vi "Init Events.vi"(8 "error in (no error)":errorcluster, 11 "DbgTimers in":refnum<class "DbgTimers.lvclass">) -> (0 "error out":errorcluster, 3 "DbgTimers out":refnum<class "DbgTimers.lvclass">)   [LabVIEW 2017, in "DbgTimers.lvclass"]
doc: "Developed by Kevin Thompson\nkevin@thompsonengineering.net\n\nCopyright 2018-2020\nThompson Engineering, LLC"
uses:
  DbgTimers.lvclass
  Ichor_Common/DataTypes/TD Async CmdMsg EventData--cluster.ctl
  DbgTimers.lvclass/DbgTimers.ctl
  Accessors/Get PublicEvents.vi
  Accessors/Set PublicEvents.vi
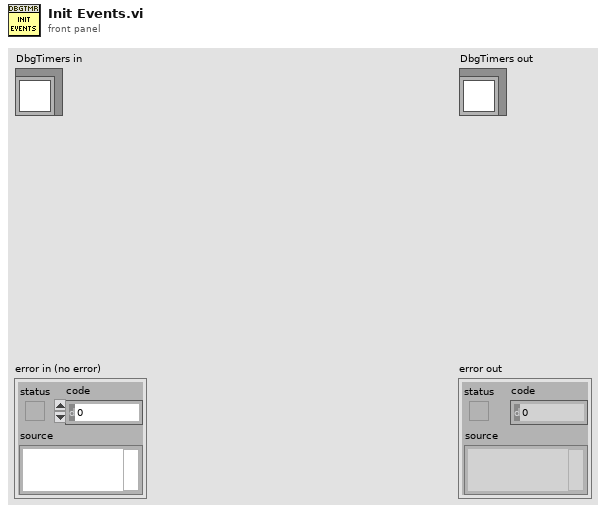
[diagram p1: front panel]
types:
  T1 = typedef "TD Async CmdMsg EventData--cluster.ctl" = cluster{"Time Stamp":timestamp, "CmdMsg":string, "vData":variant}
  T2 = typedef "DbgTimers.lvclass/Public Events--cluster.ctl" = cluster{"DbgTimers.AsyncCmd Event":refnum<user-event>, "DbgTimers.AsyncMsg Event":refnum<user-event>, "stop process":refnum<user-event>}
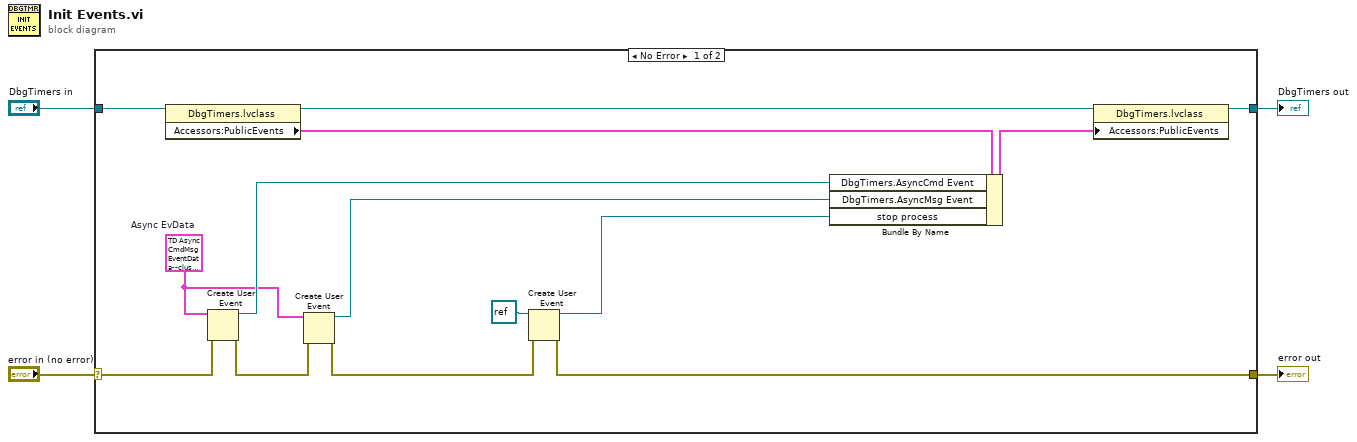
[diagram p0: block diagram]
diagram:
  n1 = case shown="No Error" "error in (no error)" {
    selector: "error in (no error)" -> [w9 w20]
    tunnel: [w10 w20] -> w3
    tunnel: [w18 w19] -> w1
    tunnel: "DbgTimers in" -> [w17 w19]
    frame No Error {
      w6 = T1 {"Time Stamp"=timestamp(0 s since 1904-01-01), "CmdMsg"="", "vData"=variant}  # Async EvData
      n2 = property class="DbgTimers.lvclass"(reference=w17) -> (reference out=w16:refnum<class "DbgTimers.lvclass">, "Accessors:PublicEvents"=w15:T2)  [unwired: 1 in, 1 out]
      n3 = Create User Event(user event datatype=w6, error in=w9) -> (user event=w11:refnum<user-event>, error out=w8:errorcluster)
      n4 = Create User Event(user event datatype=w6, error in=w8) -> (user event=w5:refnum<user-event>, error out=w7:errorcluster)
      n5 = Create User Event(user event datatype=refnum<notifier> refnum ("notifier out"), error in=w7) -> (user event=w12:refnum<user-event>, error out=w10:errorcluster)
      n6 = Bundle By Name(cluster=w15, "DbgTimers.AsyncCmd Event"=w11, "DbgTimers.AsyncMsg Event"=w5, "stop process"=w12) -> (w14:T2)
      n7 = property class="DbgTimers.lvclass"(reference=w16, "Accessors:PublicEvents"=w14) -> (reference out=w18:refnum<class "DbgTimers.lvclass">)  [unwired: 1 in, 1 out]
    }
    frame Error {
    }
  }
  "error out" <- w3
  "DbgTimers out" <- w1
